vi "plot_interferogram.vi"(0 "reference":refnum<class "OSA.lvclass">, 4 "autoScale Y":bool, 5 "error in (no error)":errorcluster, 7 "skip":bool, 9 "error rangeViolation":bool) -> (14 "duplicate reference":refnum<class "OSA.lvclass">, 19 "error out":errorcluster)   [LabVIEW 2010, in "OSA.lvclass"]
doc: "This will write a plot in an intensity graph if corresponding reference has been provided to init.vi. A compatible graph to copy can be found in the tree.vi."
uses:
  OSA.lvclass
  typeDef/xVal_option.ctl
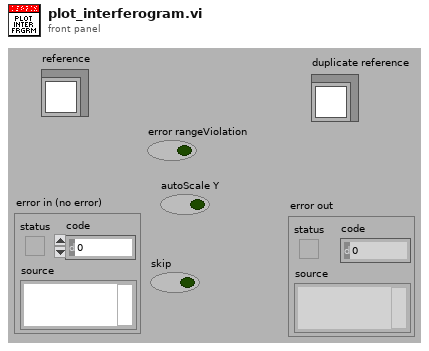
[diagram p1: front panel]
types:
  T1 = typedef "OSA.lvclass/xVal_option.ctl" = enum16{"MIN_MAX", "ARRAY"}
  T2 = cluster{"length":u32, "X min":sgl, "X max":sgl, "X_VAL_OPTIONS":T1}
  T3 = enum16{"get", "init", "set interferogram", "set spectrum", "cleanUp"}
  T4 = typedef "OSA.lvclass/ObjectAttributes.ctl" = cluster{"Stop":bool, "dataType":T5, "spectrometerIdx":u16, "buffer size interferogram":i32, "interferogram":cluster{"new":bool, "plot_x_ min":sgl, "plot_x_max":sgl, "plot_y_min":sgl, "plot_y_max":sgl, "Graph Intrfrgrm":T6, "timeStamp":u32, "signal (%)":dbl, "traces":cluster{"idx":u32, "broadBand":bool, "monoChromatic":bool, "peakToPeakSignal":dbl, "peakToPeakPos":dbl}[], "traces idx last":i32}, "spectrum":cluster{"new":bool, "plot_x_min":sgl, "plot_x_max":sgl, "plot_unit_x":T7, "plot_unit_y":T8, "plot_y_min":sgl, "plot_y_max":sgl, "Graph Spectrum":T6, "timeStamp":u32, "X_VAL_OPTIONS":enum16{"MIN_MAX", "ARRAY"}, "traces":cluster{"idx":u32}[], "traces idx last":i32}, "Thorlabs_OSA_64.lvclass:queue_action.ctlqueue ref":refnum<queue>, "action":T9, "plot zoom step":dbl, "buffer semaphore":T10, "acq stopped":bool, "dataType active":T5, "temperature (degr C)":sgl, "pressure (hPa)":sgl, "rel humidity (%)":sgl, "settings":cluster{"resolution":u16, "sensitivity":u16, "Average":bool, "average nr":u32, "apodisation":T11, "acq delay (ms)":u32, "airMesure":T12, "wmtr on":bool, "intfgrm_smooth_width":u16, "intfgrm_smooth_nrOfPasses":u16, "intfgrm_smooth":T13, "phaseCorrection":T14, "zeroFill":u8, "spectr_smooth":T13, "spectr_smooth_width":u16, "spectr_smooth_nrOfPasses":u16, "resolution (/cm)":sgl, "REF wavelength, (nm)":dbl, "gain_idx":u16, "gainAuto":bool, "gain_relative":dbl, "PD sensitivity mode":T15, "PD senseMode implemented":bool, "SensorTemperature implemented":bool, "SensorPressure implemented":bool, "SensorHumidity implemented":bool}, "peaks position":sgl[], "peaks width":sgl[], "peaks height":sgl[], "peaks max nr":u32, "peaks latest nr":i32, "peaks new":bool, "power":dbl, "power new":bool, "path":string, "wavelength (WNr)":dbl, "wavelength new":bool, "buffer size spectrum":i32, "status":string, "VI reference":refnum<vi>, "funcPointer":u64, "libraryPointer":u64, "singleAcquisition":bool, "coherenceLength (cm)":dbl, "coherenceLength new":bool, "spectrometer model":string, "spectrometer serial nr":string, "peaks thld left":sgl[], "peaks thld right":sgl[], "coherenceLength error (cm)":dbl, "ADC bits":u16, "peaks position centroid":sgl[], "peaks height centroid":sgl[], "OSA series":T16, "channel index spectrum":u16, "spectrometer rangeLow, (/cm)":dbl, "spectrometer rangeHigh, (/cm)":dbl, "channel index interferogram":u16}
  T5 = typedef "OSA.lvclass/acq_dataType.ctl" = enum16{"none", "interferogram", "spectrum"}
  T6 = typedef "OSA.lvclass/graph_intensity.ctl" = refnum<vi>
  T7 = typedef "OSA.lvclass/spectrum_x_unit.ctl" = enum16{"wavenr/cm", "THz", "eV", "nm_air", "nm_vac"}
  T8 = typedef "OSA.lvclass/y_unit.ctl" = enum16{"ADC counts", "dBm pwr absolute", "dBm pwr density", "mW pwr absolute", "mW pwr density"}
  T9 = typedef "OSA.lvclass/queue_action.ctl" = enum16{"none", "stop", "GUI_plotInterferogram", "GUI_plotSpectrum", "GUI_plotInterferogramRescale", "GUI_plotSpectrumRescale", "GUI_plotInterferogramReset", "GUI_plotSpectrumReset", "GUI_plotInterferogramAutoScaleY", "GUI_plotSpectrumAutoScaleY", "GUI_plotInterferogramZoomOut", "GUI_plotSpectrumZoomOut", "GUI_plotInterferogramPane", "GUI_plotSpectrumPane", "GUI_plotInterferogramZoomMouse", "GUI_plotSpectrumZoomMouse", "ENVIRONMENT temperature", "ENVIRONMENT pressure", "MODE_resolution set", "MODE_resolution get", "MODE_sensitivity set", "MODE_sensitivity get", "MODE_PDTemperature set", "MODE_PDTemperature get", "REBOOT/RESET firmware", "ACQASYNC_acquireSingleSpectrum", "ACQASYNC_continuous start", "ACQASYNC_continuous stop\n", "ACQASYNC_get last interferogram", "ACQASYNC_get last spectrum", "ACQASYNC_get last waveNr", "ACQOPT_interferogram smoothing set", "ACQOPT_interferogram smoothing get", "ACQOPT_spectrum smoothing set", "ACQOPT_spectrum smoothing get", "ACQOPT_apodisation type set", "ACQOPT_apodisation type get", "ACQOPT_phase correction type set", "ACQOPT_phase correction type get", "ACQOPT_acqIntervall_set", "ACQOPT_acqIntervall_get", "ACQOPT_average spectrum set", "ACQOPT_average spectrum get", "ACQOPT_rolling average set", "ACQOPT_rolling average get", "ACQOPT_zero fill factor set", "ACQOPT_zero fill factor get", "ACQOPT_cycle counting set", "ACQOPT_cycle counting get", "ACQOPT_air measure option set", "ACQOPT_air measure option get", "ACQOPT_gainLevel auto get", "ACQOPT_gainLevel auto set", "ACQOPT_gainLevel get", "ACQOPT_gainLevel set", "ACQOPT_getAll", "INSTRUMENT_PROPERTY_range_WaveNr_min", "INSTRUMENT_PROPERTY_range_WaveNr_max", "INSTRUMENT_PROPERTY_reference_wavelength_cm^-1", "INSTRUMENT_PROPERTY_samplesPerRefPeriod", "INSTRUMENT_PROPERTY_resolution_waveNrPercm", "INSTRUMENT_PROPERTY_availableGainLevels", "INSTRUMENT_PROPERTY_status", "CONVERT", "ANALYSE_POWER", "ANALYSE_PEAKS", "ANALYSE_WAVELENGTH", "ANALYSE_SPECTRUM", "ANALYSE_INTERFEROGRAM", "ANALYSE_COHERENCE_LENGTH", "MATH", "MATH_power", "MATH_peaks", "FILE", "miscellaneous"}
  T10 = typedef "Semaphore RefNum" = refnum<k1>
  T11 = typedef "OSA.lvclass/apodisation.ctl" = enum16{"NONE", "NORTON_BEER_WEAK", "NORTON_BEER_MEDIUM", "NORTON_BEER_STRONG", "TRIANGULAR", "COSINE", "HANN", "HAMMING", "BLACKMANHARRIS3", "BLACKMANHARRIS4", "GAUSSIAN"}
  T12 = typedef "OSA.lvclass/airMeasure.ctl" = enum16{"TEMPERATURE", "PRESSURE"}
  T13 = typedef "OSA20X_misc.lvlib/interferogram_smoothing.ctl" = enum16{"NONE", "BINOMIAL", "SAVITSKY_GOLAY", "FOURIER", "MOVING_AVERAGE", "GAUSSIAN"}
  T14 = typedef "OSA.lvclass/phaseCorrection.ctl" = enum16{"NONE", "MERTZ", "FORMAN", "MERTZ_FILE", "FORMAN_FILE", "FUTURE COMP."}
  T15 = typedef "OSA20X_misc.lvlib/PDTemperatureMode.ctl" = enum16{"cool: better sensitivity/noise floor", "warm: extended wl range"}
  T16 = typedef "OSA.lvclass/OSA_series.ctl" = enum16{"OSA200", "OSA300", "UNKNOWN"}
  T17 = cluster{"length":u32, "X min (cm)":sgl, "X max (cm)":sgl, "saturated":bool, "broadband":bool, "isMonoChromatic":bool, "peakToPeak, (counts)":dbl, "peakToPeak position (cm)":dbl, "samplesPerRefPeriod":i32}
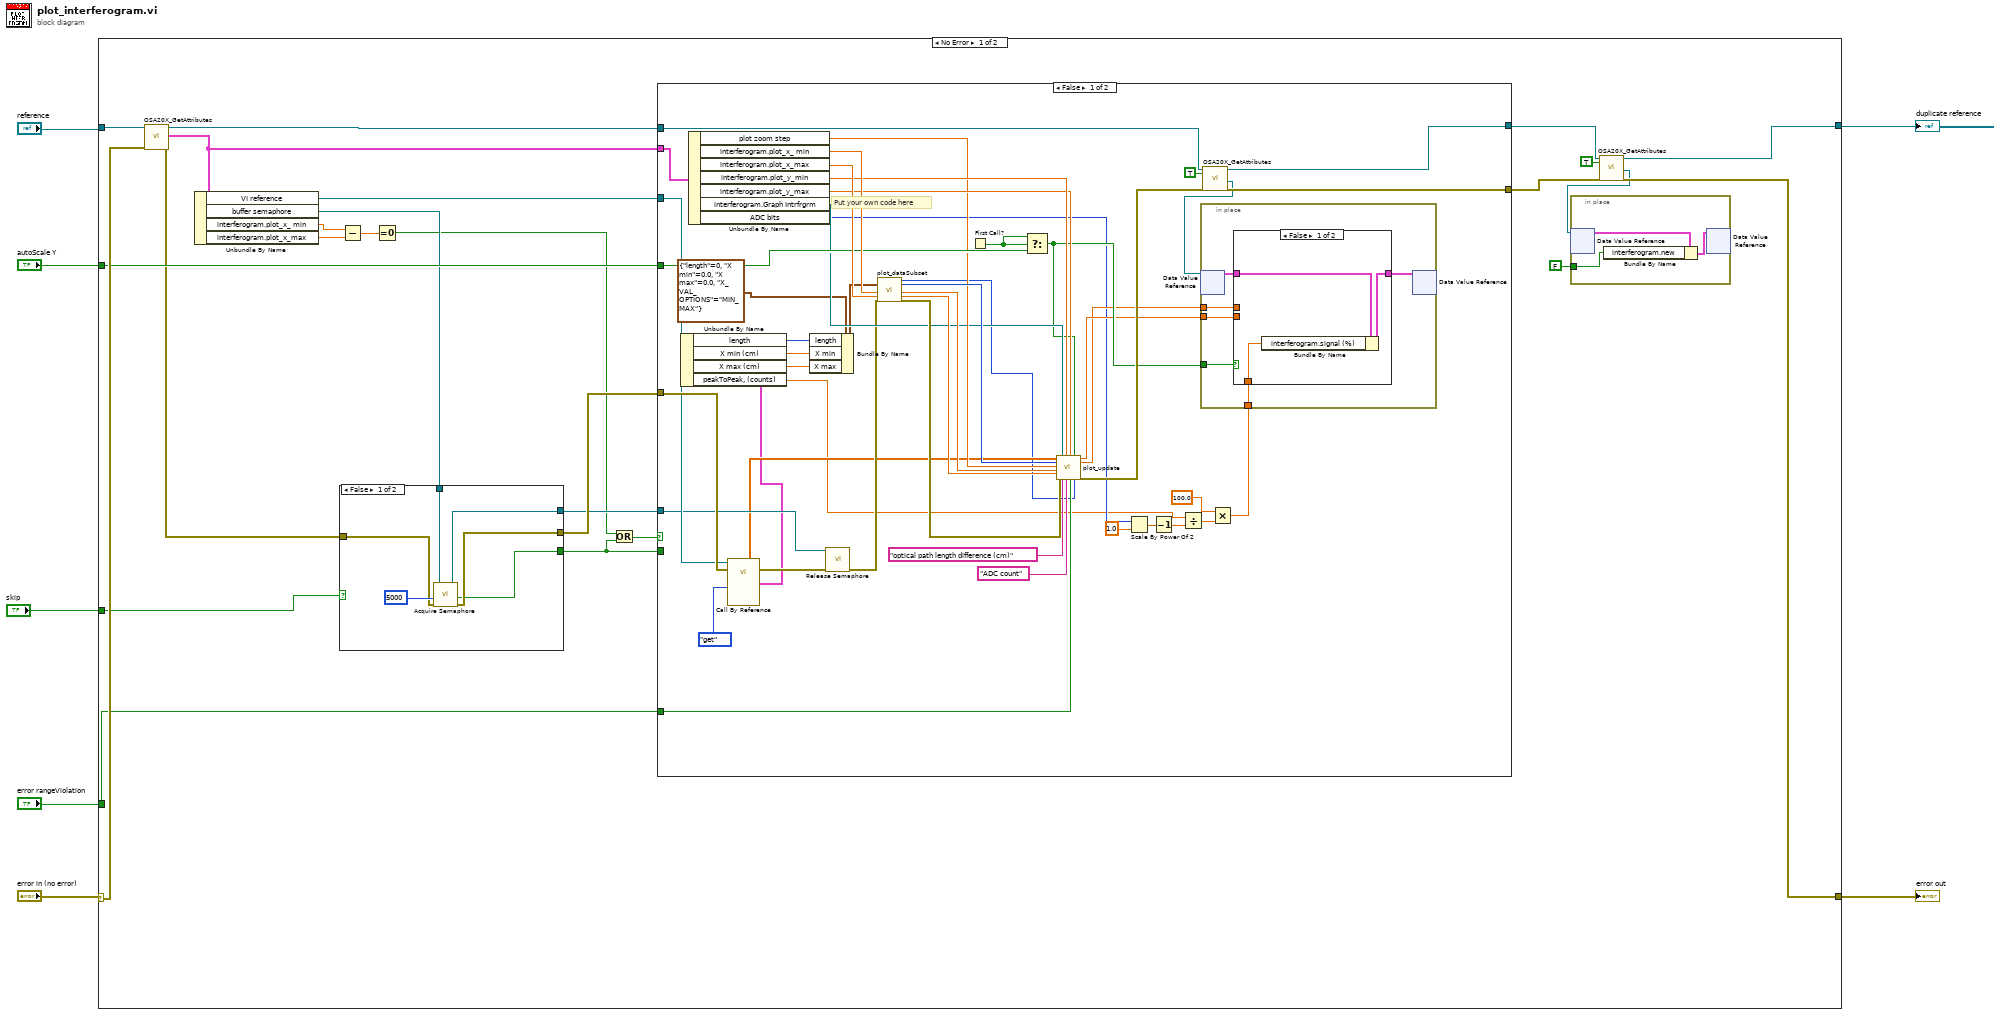
[diagram p0: block diagram]
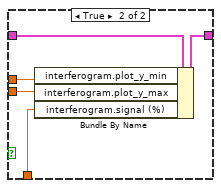
[diagram p3: hidden frame]
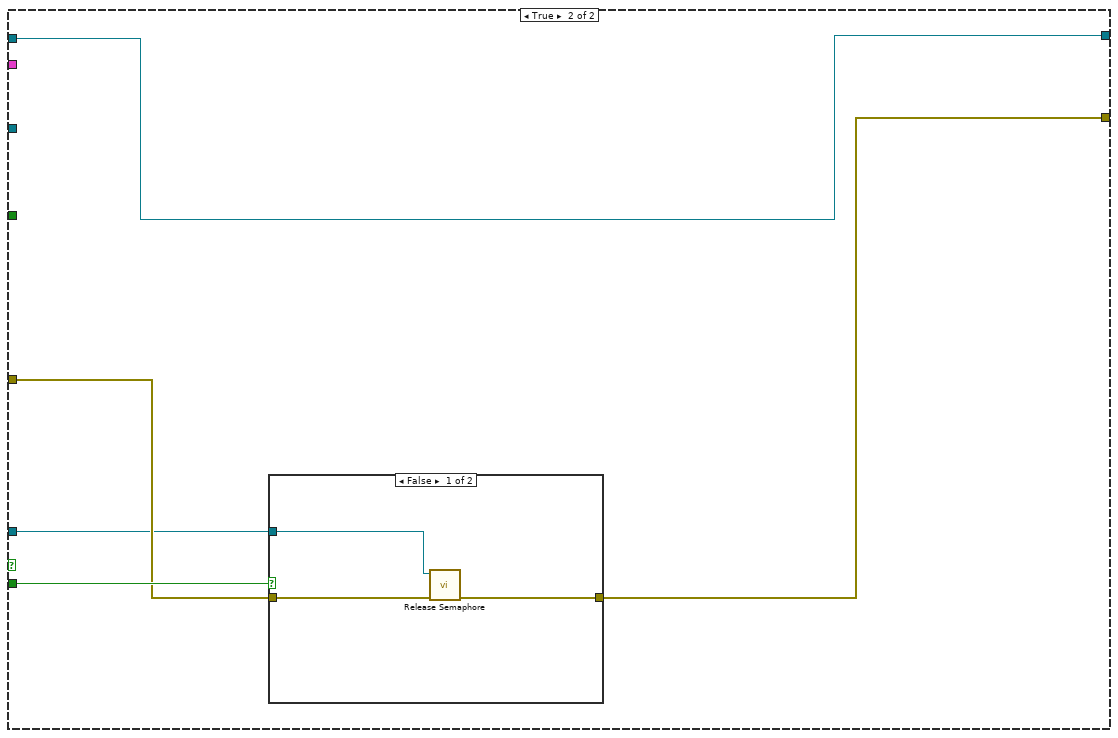
[diagram p4: hidden frame]
diagram:
  n1 = case shown="No Error" "error in (no error)" {
    selector: "error in (no error)" -> [w31 w115]
    tunnel: [w25 w115] -> w7
    tunnel: "reference" -> [w32 w116]
    tunnel: [w27 w116] -> w4
    tunnel: "error rangeViolation" -> [w30 _]
    tunnel: "autoScale Y" -> [w29 _]
    tunnel: "skip" -> [w19 _]
    frame No Error {
      n2 = call "OSA20X_GetAttributes.vi"("reference in"=w32, "error in (no error)"=w31) -> ("reference out"=w21:refnum<class "OSA.lvclass">, "Data"=w10:T4, "error out"=w20:errorcluster)  [unwired: 14 in, 1 out]
      n3 = Unbundle By Name(w10) -> ("VI reference"=w22:refnum<vi>, "buffer semaphore"=w24:T10, "interferogram.plot_x_ min"=w15:sgl, "interferogram.plot_x_max"=w14:sgl)
      n4 = case shown="False" w19 {
        selector: w19 -> [_ w43]
        tunnel: w24 -> [w41 w42]
        tunnel: [w39 w44] -> w23
        tunnel: w20 -> [w38 w44]
        tunnel: [w37 w43] -> w12
        tunnel: [w36 w42] -> w18
        frame False {
          n5 = call <vilib>:"Acquire Semaphore.vi"("error in (no error)"=w38, "ms timeout (-1)"=5000, "semaphore"=w41) -> ("error out"=w39:errorcluster, "timed out"=w37:bool, "semaphore out"=w36:T10)  [unwired: 2 in]
        }
        frame True {
        }
      }
      n6 = Subtract(x=w15, y=w14) -> (x-y=w13:sgl)
      n7 = Equal To 0?(x=w13) -> (x = 0?=w17:bool)
      n8 = Or(x=w17, y=w12) -> (x .or. y?=w16:bool)
      n9 = case shown="False" w16 {
        tunnel: w21 -> [w89 w110]
        tunnel: [w88 w110] -> w28
        tunnel: [w86 w106] -> w26
        tunnel: w10 -> [w85 _]
        tunnel: w23 -> [w70 w108]
        tunnel: w30 -> [w78 _]
        tunnel: w29 -> [w74 _]
        tunnel: w22 -> [w69 _]
        tunnel: w18 -> [w68 w107]
        tunnel: w12 -> [_ w109]
        frame False {
          # "Put your own code here"
          n10 = Unbundle By Name(w85) -> ("plot zoom step"=w73:dbl, "interferogram.plot_x_ min"=w84:sgl, "interferogram.plot_x_max"=w83:sgl, "interferogram.plot_y_min"=w77:sgl, "interferogram.plot_y_max"=w76:sgl, "interferogram.Graph Intrfrgrm"=w72:T6, "ADC bits"=w54:u16)
          n11 = call-by-ref "?"(reference=w69, error in=w70, "action"=T3."get") -> (error out=w67:errorcluster, "interferogram"=w65:sgl[], "interferogram prop set"=w58:T17)  [unwired: 14 in, 4 out]
          n12 = Unbundle By Name(w58) -> ("length"=w57:u32, "X min (cm)"=w56:sgl, "X max (cm)"=w55:sgl, "peakToPeak, (counts)"=w51:dbl)
          n13 = Bundle By Name(cluster=T2 {"length"=0, "X min"=0.0, "X max"=0.0, "X_VAL_OPTIONS"=enum."MIN_MAX"} ("spectrum property"), "length"=w57, "X min"=w56, "X max"=w55) -> (w45:T2)
          n14 = call <vilib>:"Release Semaphore.vi"("error in (no error)"=w67, "semaphore"=w68) -> ("error out"=w66:errorcluster)  [unwired: 4 in, 1 out]
          n15 = call "plot_dataSubset.vi"("spectrum property"=w45, "zoom range low"=w84, "zoom range high"=w83, "error in (no error)"=w66) -> ("idx start"=w64:i32, "length"=w82:i32, "X min actual"=w81:sgl, "X max actual"=w80:sgl, "error out"=w79:errorcluster)  [unwired: 11 in]
          n16 = First Call?() -> (First Call?: T/F=w75:bool)
          n17 = Select(t=w75, s=w75, f=w74) -> (s? t:f=w61:bool)
          n18 = call "plot_update.vi"("data"=w65, "data length"=w82, "x zoom factor"=w73, "X range min"=w81, "X range max"=w80, "error in (no error)"=w79, "graph ref"=w72, "X Scale.Name Label.Text"="optical path length difference (cm)", "y min value"=w77, "Y Scale.Name Label.Text"="ADC count", "y max value"=w76, "error rangeViolation"=w78, "autoScale Y"=w61, "data idxStart"=w64) -> ("dataVal max"=w60:sgl, "dataVal min"=w59:sgl, "error out"=w87:errorcluster)  [unwired: 3 in]
          n19 = Scale By Power Of 2(n=w54, x=1.0) -> (x*2^n=w52:dbl)
          n20 = Decrement(x=w52) -> (x-1=w47:dbl)
          n21 = Divide(x=w51, y=w47) -> (x/y=w50:dbl)
          n22 = call "OSA20X_GetAttributes.vi"("reference in"=w89, "OnlyGetDvrReference(False)"=TRUE, "error in (no error)"=w87) -> ("reference out"=w88:refnum<class "OSA.lvclass">, "DataRef"=w62:refnum<data-value>, "error out"=w86:errorcluster)  [unwired: 13 in, 1 out]
          n23 = Multiply(x=100.0, y=w50) -> (x*y=w48:dbl)
          n24 = in-place {
            in-place-border: w61 -> [w97]
            in-place-border: w60 -> [w95]
            in-place-border: w59 -> [w94]
            in-place-border: w48 -> [w92]
            n25 = in-place-dvr #1(w62) -> (w96:T4)  [unwired: 1 out]
            n26 = case shown="False" w97 {
              tunnel: w96 -> [w100 w104]
              tunnel: [w99 w105] -> w93
              tunnel: w95 -> [_ w103]
              tunnel: w94 -> [_ w102]
              tunnel: w92 -> [w98 w101]
              frame False {
                n27 = Bundle By Name(cluster=w100, "interferogram.signal (%)"=w98) -> (w99:T4)
              }
              frame True {
                n28 = Bundle By Name(cluster=w104, "interferogram.plot_y_min"=w102, "interferogram.plot_y_max"=w103, "interferogram.signal (%)"=w101) -> (w105:T4)
              }
            }
            n29 = in-place-dvr #1(w93) -> ()  [unwired: 2 out]
          }
        }
        frame True {
          n30 = case shown="False" w109 {
            tunnel: w108 -> [w113 w114]
            tunnel: w107 -> [w112 _]
            tunnel: [w111 w114] -> w106
            frame False {
              n31 = call <vilib>:"Release Semaphore.vi"("error in (no error)"=w113, "semaphore"=w112) -> ("error out"=w111:errorcluster)  [unwired: 4 in, 1 out]
            }
            frame True {
            }
          }
        }
      }
      n32 = call "OSA20X_GetAttributes.vi"("reference in"=w28, "OnlyGetDvrReference(False)"=TRUE, "error in (no error)"=w26) -> ("reference out"=w27:refnum<class "OSA.lvclass">, "DataRef"=w9:refnum<data-value>, "error out"=w25:errorcluster)  [unwired: 13 in, 1 out]
      n33 = in-place {
        in-place-border: FALSE ("dataNewIntrfrgrm") -> [w34]
        n34 = in-place-dvr #2(w9) -> (w35:T4)  [unwired: 1 out]
        n35 = Bundle By Name(cluster=w35, "interferogram.new"=w34) -> (w33:T4)
        n36 = in-place-dvr #2(w33) -> ()  [unwired: 2 out]
      }
    }
    frame Error {
      # "Error"
    }
  }
  "error out" <- w7
  "duplicate reference" <- w4
